vi "dblvector_filtave.vi"(9 "Eldobandó [%]":dbl=40.0 min=0.0 max=50.0, 11 "Mérési adatok":dbl[](array[numeric])=[0.08666794019762783, 0.08601728999766332, 0.0864271996183335, 0.08608886151743325, 0.08607584851379788, 0.08610187452108677, 0.0861213940266011, 0.0860498225065816, 0.08601728999766332, 0.08610187452108677, 0.08611488752475846, 0.08608235501561329, 0.0861734460415058, 0.08600427699412777, 0.08606283551018067, 0.08616043303775238, 0.08616693953962681, 0.08615392653588247, 0.0861734460415058, 0.08636213459797418, 0.08623200455862118, 0.0861734460415058, 0.08619296554717003, 0.08615392653588247, 0.08614091353215629, 0.08625152406440813, 0.08621899155478593, 0.08618645904527741, 0.08619947204906718, 0.08645973212868403, 0.0861734460415058, 0.08621248505287515, 0.0861734460415058, 0.0861734460415058, 0.08618645904527741, 0.08616043303775238, 0.08627755007218772, 0.08617995254338934, 0.08619947204906718, 0.08621899155478593, 0.0862254980567013, 0.08600427699412777, 0.08621248505287515, 0.08623200455862118, 0.0859261989732952, 0.08539266584836862, 0.08616693953962681, 0.08545773086197897, 0.08584812095311502, 0.08607584851379788, 0.08610187452108677, 0.08610187452108677, 0.08578956243840764, 0.0861213940266011, 0.0861213940266011, 0.08612790052844829, 0.0859652379836299, 0.08625152406440813, 0.08613440703030002, 0.0861213940266011, 0.08611488752475846, 0.08627104357023599, 0.08610838102292034, 0.08618645904527741, 0.08614091353215629, 0.08614742003401712, 0.08614091353215629, 0.08578305593679611, 0.0862254980567013, 0.08613440703030002, 0.08612790052844829, 0.08614742003401712, 0.08633610858995795, 0.08615392653588247, 0.0861734460415058, 0.08616043303775238, 0.0861734460415058, 0.08666143369540256, 0.08618645904527741, 0.08625803056634619, 0.0862059785509689, 0.08619947204906718, 0.08706483684202262, 0.08615392653588247, 0.086284056574144, 0.0862450175624746, 0.08621899155478593, 0.0862059785509689, 0.0870323043295454, 0.08586764045809894, 0.08627755007218772, 0.0862254980567013, 0.0862254980567013, 0.0862254980567013, 0.08533410733650425, 0.08653781015399033, 0.08621248505287515, 0.08625803056634619, 0.0862254980567013, 0.08595222498016687, 0.08645322562660482, 0.08638165410403414, 0.08626453706828882, 0.08626453706828882, 0.08626453706828882, 0.0861213940266011, 0.08616693953962681, 0.08626453706828882, 0.086284056574144, 0.0862450175624746, 0.08626453706828882, 0.08614742003401712, 0.08621899155478593, 0.08625152406440813, 0.08627104357023599, 0.08626453706828882, 0.08706483684202262, 0.08612790052844829, 0.08627755007218772, 0.08627104357023599, 0.0862450175624746, 0.08627755007218772, 0.0862059785509689, 0.08630357608004009, 0.08627104357023599, 0.08625152406440813, 0.08626453706828882, 0.08625152406440813, 0.08651829064760218, 0.086284056574144, 0.0862385110605456, 0.08627755007218772, 0.08625152406440813, 0.08634261509195519, 0.0862450175624746, 0.08625803056634619, 0.0862450175624746, 0.08626453706828882, 0.0862450175624746, 0.08619947204906718, 0.0862385110605456, 0.0862450175624746, 0.08625152406440813, 0.08623200455862118, 0.08686313526651203, 0.08709086285208703, 0.087058330339518, 0.08704531733452252, 0.08666794019762783, 0.08694771979764135, 0.0870323043295454, 0.08697374580737542, 0.08695422630006798, 0.08697374580737542, 0.08694771979764135, 0.08699977181718288, 0.08694771979764135, 0.0868891612760078, 0.08692169378798062, 0.08690868078317775, 0.086882654773627, 0.08693470679280181, 0.08699326531472412, 0.08694771979764135, 0.08727304492459627, 0.08671348571333262, 0.08677204423385369, 0.08679807024309312, 0.08678505723846426, 0.08676553773155528, 0.08636213459797418, 0.08668095320209206, 0.08677204423385369, 0.08679807024309312, 0.08676553773155528, 0.08658986217122618, 0.08659636867340119, 0.08653781015399033, 0.08647925163494903, 0.08645322562660482, 0.08642069311627706, 0.08652479714972701, 0.08626453706828882, 0.08630357608004009, 0.08626453706828882, 0.086284056574144, 0.08617995254338934, 0.08573751042564201, 0.08644021262246004, 0.08612790052844829, 0.08616043303775238, 0.08617995254338934, 0.08447524920423201, 0.08642069311627706, 0.08601728999766332, 0.08626453706828882, 0.08614091353215629, 0.08619947204906718, 0.08658335566905571, 0.0858546274547718]) -> (3 "Szûrt átlag":dbl=0.08628641518298938)   [LabVIEW 2014]
doc: "Kiszámítja az 1DArray elemeinek átlagértékét. (Average)"
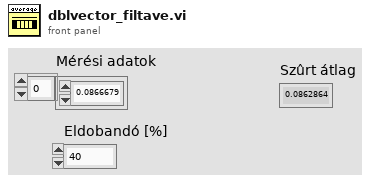
[diagram p1: front panel]
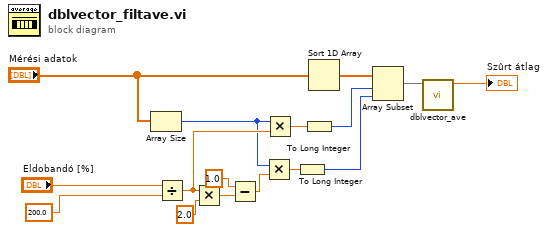
[diagram p0: block diagram]
diagram:
  n1 = Array Size(array="Mérési adatok") -> (size(s)=w6:i32)
  n2 = Divide(x="Eldobandó [%]", y=200.0) -> (x/y=w7:dbl)
  n3 = Multiply(x=w7, y=2.0) -> (x*y=w9:dbl)
  n4 = Subtract(x=1.0, y=w9) -> (x-y=w5:dbl)
  n5 = Multiply(x=w6, y=w5) -> (x*y=w4:dbl)
  n6 = Multiply(x=w6, y=w7) -> (x*y=w3:dbl)
  n7 = To Long Integer(number=w4) -> (32bit integer=w1:i32)
  n8 = To Long Integer(number=w3) -> (32bit integer=w2:i32)
  n9 = Sort 1D Array(array="Mérési adatok") -> (sorted array=w15:dbl[])
  n10 = Array Subset(array=w15, index=w2, length=w1) -> (w14:dbl[])
  n11 = call "dblvector_ave.vi"("1DArray"=w14) -> ("Average"=→"Szûrt átlag":dbl)  [unwired: 10 in]
